vi "Simple DC Motor Control_test.vi"() -> ()   [LabVIEW 2013]
uses:
  <vilib>/measure/mascope.llb/Amplitude and Levels N chan.vi
  <vilib>/measure/NI_MAPro.lvlib
panel:
  in  "Tab Control":enum32{"DC Motor"}(tab)
  in  "STOP":bool
  out "RPM-Counterclockwise":dbl
  out "Encoder Input - Counterclockwise":dynamicdata(graph)
  out "Encoder Input - Clockwise":dynamicdata(graph)
  in  "Direction":u16(ring) items=["Clockwise", "Counter-Clockwise"]
  out "RPM-Clockwise":dbl
  in  "STOP":bool
  # "DC Motor Controller"
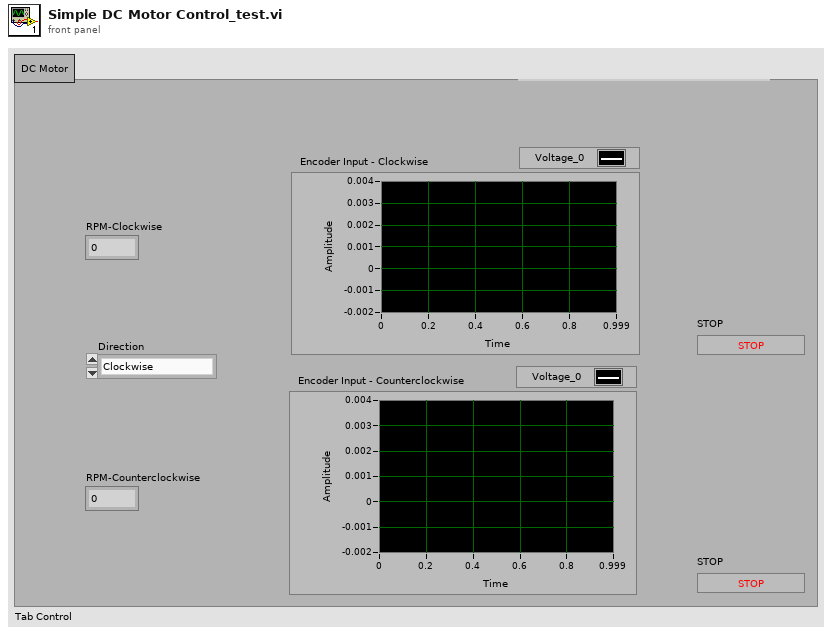
[diagram p1: front panel]
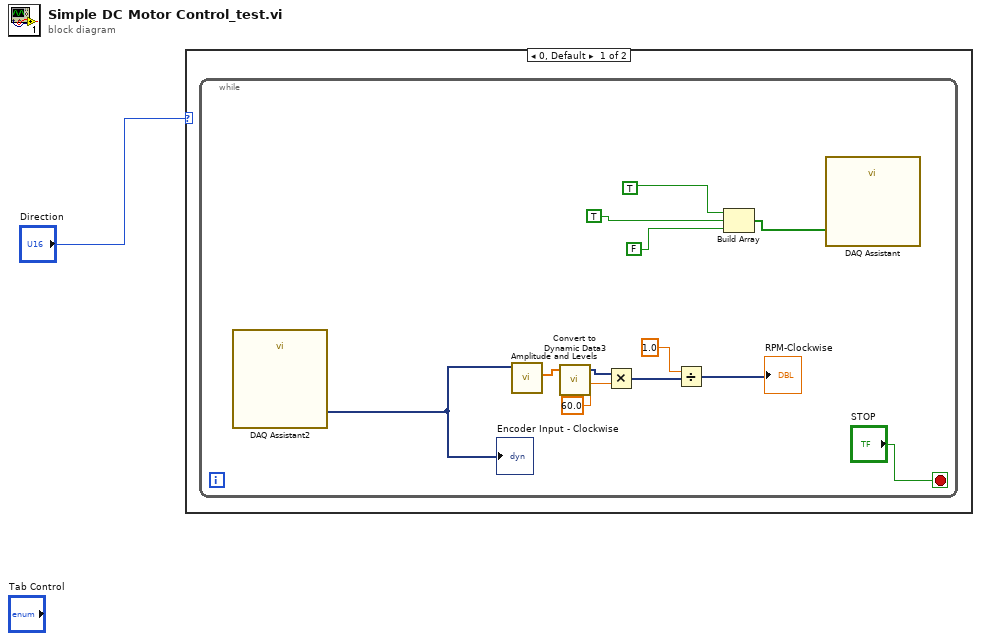
[diagram p0: block diagram]
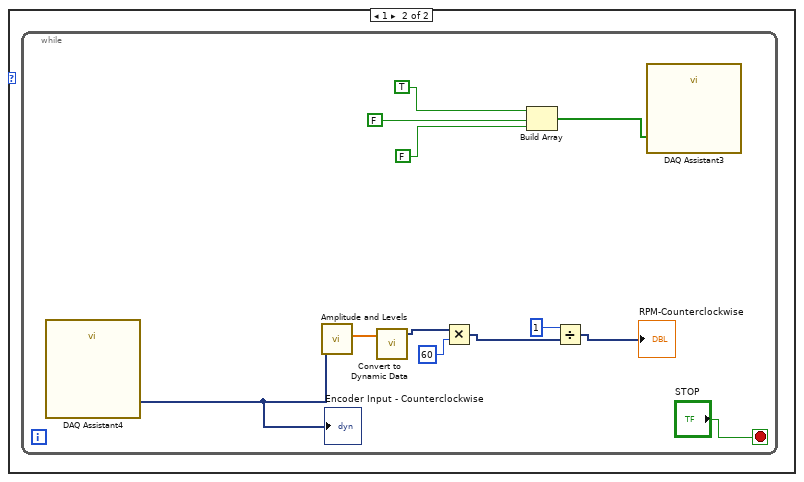
[diagram p2: hidden frame]
diagram:
  n1 = case shown="0, Default" "Direction" {
    frame 0, Default {
      n2 = while {
        stop <- "STOP" stop-if-true
        n3 = call "DAQ Assistant2"() -> ("data"=w2:dynamicdata)  [unwired: 16 in, 3 out]
        "Encoder Input - Clockwise" <- w2
        n4 = call-poly <vilib>:"Amplitude and Levels.vi"("signal(s) in"=w2) -> ("high state level"=w13:dbl[])  [unwired: 7 in, 3 out]
        n5 = call "Convert to Dynamic Data3"("Array"=w13) -> ("Dynamic Data Type"=w12:dynamicdata)  [unwired: 3 in]
        n6 = Multiply(x=w12, y=60.0) -> (x*y=w10:dynamicdata)
        n7 = Divide(x=1.0, y=w10) -> (x/y=→"RPM-Clockwise":dynamicdata)
        n8 = Build Array(TRUE ("Boolean"), TRUE, FALSE) -> (w7:bool[])
        n9 = call "DAQ Assistant"("data"=w7) -> ()  [unwired: 17 in, 2 out]
      }
    }
    frame 1 {
      n10 = while {
        stop <- "STOP" stop-if-true
        n11 = call "DAQ Assistant4"() -> ("data"=w14:dynamicdata)  [unwired: 16 in, 3 out]
        "Encoder Input - Counterclockwise" <- w14
        n12 = call-poly <vilib>:"Amplitude and Levels.vi"("signal(s) in"=w14) -> ("high state level"=w22:dbl[])  [unwired: 7 in, 3 out]
        n13 = call "Convert to Dynamic Data"("Array"=w22) -> ("Dynamic Data Type"=w21:dynamicdata)  [unwired: 3 in]
        n14 = Multiply(x=w21, y=60) -> (x*y=w24:dynamicdata)
        n15 = Build Array(TRUE, FALSE, FALSE) -> (w16:bool[])
        n16 = Divide(x=1, y=w24) -> (x/y=→"RPM-Counterclockwise":dynamicdata)
        n17 = call "DAQ Assistant3"("data"=w16) -> ()  [unwired: 17 in, 2 out]
      }
    }
  }
